vi "Setup V1.00.vi"(6 "Control Parameters Input":T1={"Grating Density"=enum."1200", "Offset"=0.0, "Save All Data in ONE file"=FALSE, "Auto Save Data"=FALSE, "Most recent saved file"=path "erererere", "Filename Prefix"="MyData", "Extension"=4, "Suffix"="", "Current Path"=path "/Volumes/DATA"} {"Extension" items=["DOS field", "\".001\",\".002\", ...", "001 (No dot)", "\".A\",\".B\", ...", "±Field", "pField nField", "Temperature", "User Defined"]; "Offset" format="%.2f"}, 7 "TempControl Input":bool[](array[boolean])=[TRUE, FALSE, FALSE, FALSE], 8 "Parameters#2 input":T2={"MaxBufferSize"=2, "Mag GPIB Address"=5, "Max Current (kA)"=36.0, "LTC-GPIB Address"="", "Temp Tolerance"=1.0} {"Temp Tolerance" format="%.2f"; "Max Current (kA)" format="%.2f"}, 9 "Parameters Input":T3={"Magnetic Field"=0.0, "Temperature"=0.0, "Exposure Time"=0.0, "Mag ID string"="", "User Name"="Albert Einstein", "Comments"="", "SaveComments?"=1, "X-Axis Unit"=1, "Delimiter"=0, "File Format"=0, "Sample Name"="Sample1"} {"File Format" items=["Macintosh (EOL: CR)", "Unix (EOL: LF)", "DOS/Windows (EOL: CR+LF)"]; "Delimiter" items=["TAB", "COMMA", "SPACE"]; "X-Axis Unit" items=["Point #", "nm", "eV", "meV", "cm-1"]; "SaveComments?" items=["Bare data only", "Saved in the Header Area", "Saved as a Parameter File"]; "Exposure Time" format="%.2f"; "Temperature" format="%.2f"; "Magnetic Field" format="%.2f"}) -> (0 "Control Parameters output":T1={"Grating Density"=enum."1200", "Offset"=0.0, "Save All Data in ONE file"=FALSE, "Auto Save Data"=FALSE, "Most recent saved file"=path "erererere", "Filename Prefix"="MyData", "Extension"=4, "Suffix"="", "Current Path"=path "/Volumes/DATA"} {"Extension" items=["DOS field", "\".001\",\".002\", ...", "001 (No dot)", "\".A\",\".B\", ...", "±Field", "pField nField", "Temperature", "User Defined"]; "Offset" format="%.2f"}, 1 "Parameters#2":T2={"MaxBufferSize"=2, "Mag GPIB Address"=5, "Max Current (kA)"=36.0, "LTC-GPIB Address"="", "Temp Tolerance"=1.0} {"Temp Tolerance" format="%.2f"; "Max Current (kA)" format="%.2f"}, 2 "TempControl":bool[](array[boolean])=[TRUE, FALSE, FALSE, FALSE], 3 "Parameters output":T3={"Magnetic Field"=0.0, "Temperature"=0.0, "Exposure Time"=0.0, "Mag ID string"="None", "User Name"="", "Comments"="", "SaveComments?"=1, "X-Axis Unit"=1, "Delimiter"=0, "File Format"=0, "Sample Name"="Sample1"} {"File Format" items=["Macintosh (EOL: CR)", "Unix (EOL: LF)", "DOS/Windows (EOL: CR+LF)"]; "Delimiter" items=["TAB", "COMMA", "SPACE"]; "X-Axis Unit" items=["Point #", "nm", "eV", "meV", "cm-1"]; "SaveComments?" items=["Bare data only", "Saved in the Header Area", "Saved as a Parameter File"]; "Exposure Time" format="%.2f"; "Temperature" format="%.2f"; "Magnetic Field" format="%.2f"}, 4 "McP off":bool=TRUE caption="McP on? output", 5 "CCD off":bool=TRUE caption="CCD on? output")   [LabVIEW 2021]
uses:
  Parameters#1.ctl
  Parameters#2.ctl
  Parameters_Control.ctl
  Globals and TypeDefs/Global Varibal Control.vi
  ExperimentLogGlobal.vi
panel:
  in  "Maximum BufferSize":u8=50 min=1 step=1
  in  "OpenUserProfile":bool
  out "Clock copy":string="1:26:45 AM"
  out "Clock":string="1:26:45 AM"
  in  "CCD on?":bool=TRUE caption="Off"
  out "CCD GPIB Address":u8=1 min=1 max=30
  in  "CCD LineSet?":bool caption="ldb,1,16,u,0,225,25,b,1,15;sdu,0,1024,1024;cl0;omrm;sron"
  in  "ChangeCounterPos?":bool
  in  "?":bool
  in  "LTC20 Cal Table?":bool
  in  "Hide?":bool
  out "GPIB Status":string
  in  "BusScan?":bool
  in  "Calibration":bool
  in  "X-Axis Unit":u16(ring)=1 items=["Point #", "nanometer (nm)", "electron volt (eV)", "Milli eV (meV)", "Wavenumber (cm-1)"]
  in  "SaveComments?":u16(ring)=1 items=["Bare data only", "Saved in the Header Area", "Saved as a Parameter File"]
  in  "Delimiter":u16(ring) items=["TAB", "COMMA", "SPACE"]
  in  "File Format":u16(ring) items=["Macintosh (EOL: CR)", "Unix (EOL: LF)", "DOS/Windows (EOL: CR+LF)"]
  in  "Max Current (kA)":dbl=36.0 caption="Maximum Current (kA)" format="%.2f"
  in  "User Name":string
  in  "Temp Tolerance":dbl=1.0 caption="Temperature Tolerance (if applicable)" format="%.2f"
  in  "LTC-GPIB Address":refnum<visa-resource-name> caption="GPIB Address"
  in  "Auto\nAdvance?":bool
  in  "Magneto\nCorrection?":bool
  in  "Mode:\nControl?":bool caption="Monitor"
  in  "LTC-20\nexist?":bool
  in  "SaveUserProfile":bool
  in  "Sample Name":string="Sample1"
  # "User Profile Panel"
  # "Magnet Control Panel"
  # "The Modem Port is reserved."
  # "Conductus LTC-20 Panel"
  # "Yes\n\nNo"
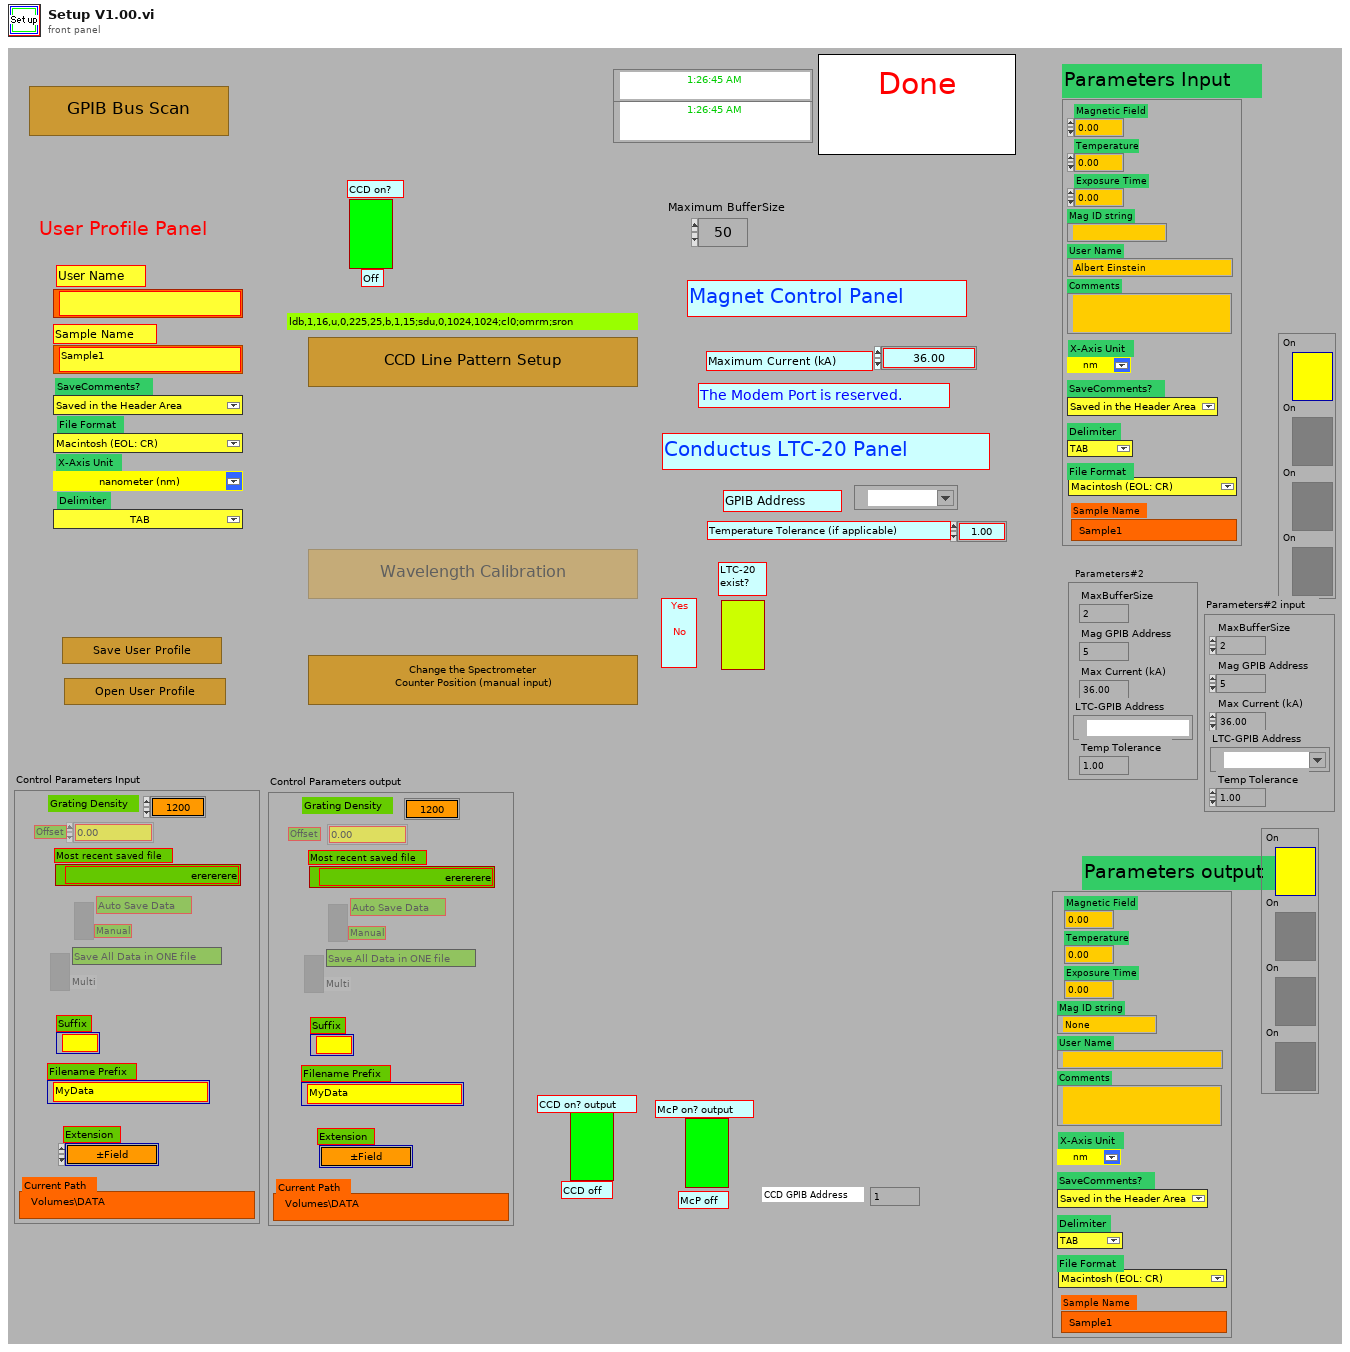
[diagram p1: front panel]
types:
  T1 = typedef "Parameters_Control.ctl" = cluster{"Grating Density":enum16{"150", "300", "600", "1200", "1800"}, "Offset":dbl, "Save All Data in ONE file":bool, "Auto Save Data":bool, "Most recent saved file":path, "Filename Prefix":string, "Extension":u16, "Suffix":string, "Current Path":path}
  T2 = typedef "Parameters#2.ctl" = cluster{"MaxBufferSize":i32, "Mag GPIB Address":i32, "Max Current (kA)":dbl, "LTC-GPIB Address":refnum<visa-resource-name>, "Temp Tolerance":dbl}
  T3 = typedef "Parameters#1.ctl" = cluster{"Magnetic Field":dbl, "Temperature":dbl, "Exposure Time":dbl, "Mag ID string":string, "User Name":string, "Comments":string, "SaveComments?":u16, "X-Axis Unit":u16, "Delimiter":u16, "File Format":u16, "Sample Name":string}
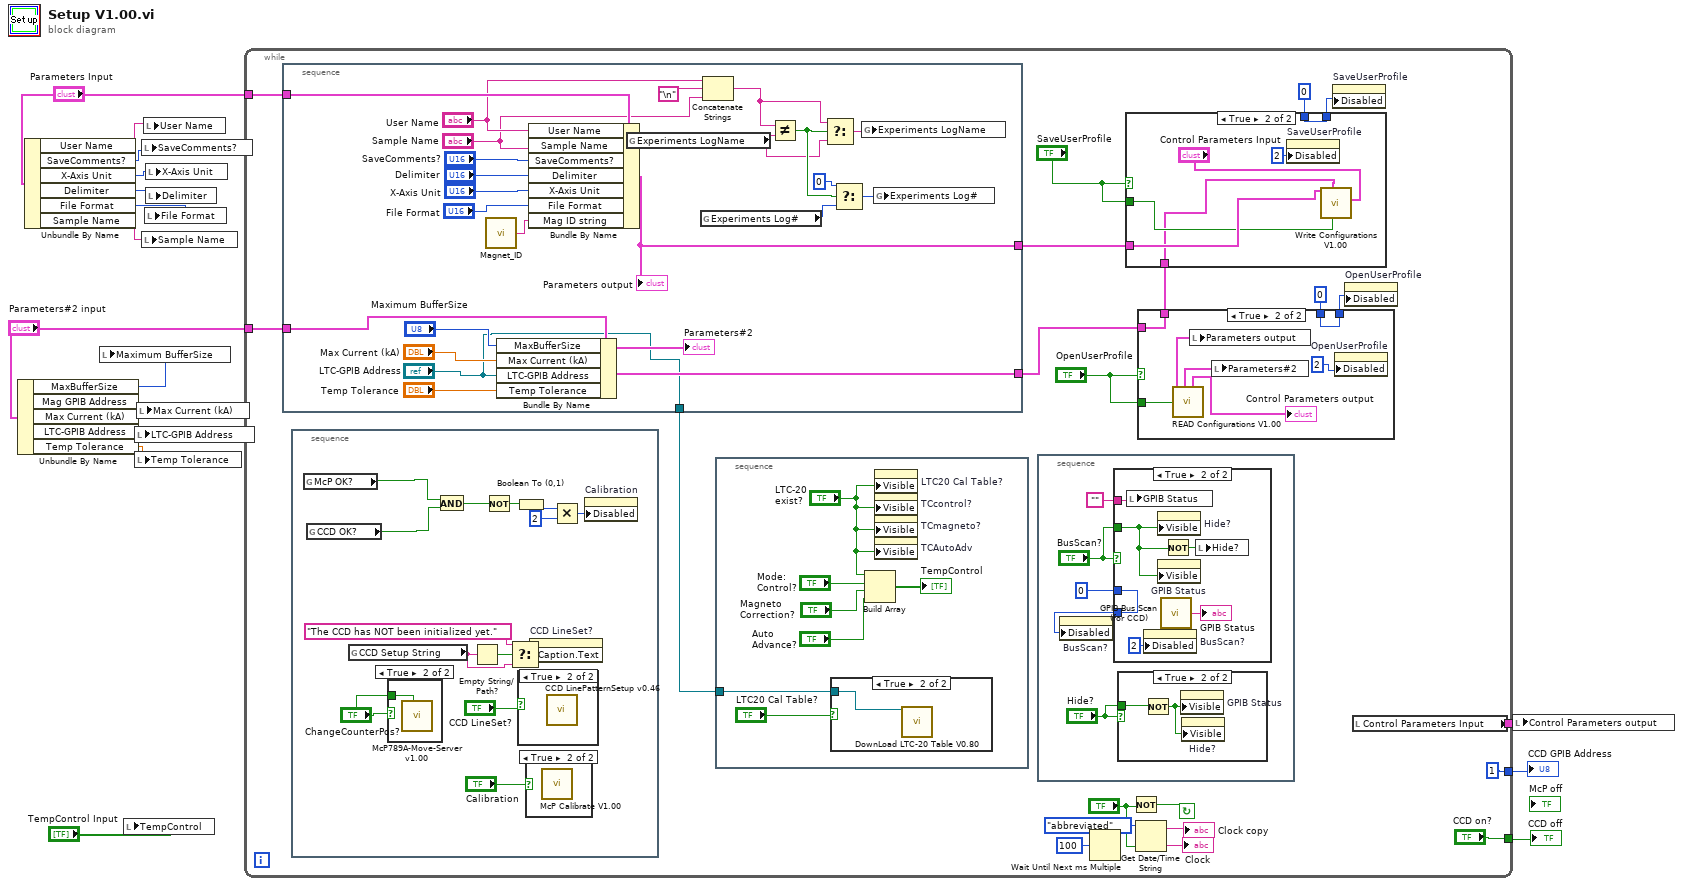
[diagram p0: block diagram]
diagram:
  n1 = Unbundle By Name("Parameters#2 input") -> ("MaxBufferSize"=w2:i32, "Max Current (kA)"=w7:dbl, "LTC-GPIB Address"=w6:refnum<visa-resource-name>, "Temp Tolerance"=w5:dbl)  [unwired: 1 out]
  n2 = Unbundle By Name("Parameters Input") -> ("User Name"=w9:string, "SaveComments?"=w10:u16, "X-Axis Unit"=w11:u16, "Delimiter"=w12:u16, "File Format"=w13:u16, "Sample Name"=w14:string)
  n3 = local write "Maximum BufferSize"(w2) -> ()
  n4 = local write "TempControl"("TempControl Input") -> ()
  n5 = local write "LTC-GPIB Address"(w6) -> ()
  n6 = local write "Temp Tolerance"(w5) -> ()
  n7 = local write "Max Current (kA)"(w7) -> ()
  n8 = local write "SaveComments?"(w10) -> ()
  n9 = local write "Sample Name"(w14) -> ()
  n10 = local write "User Name"(w9) -> ()
  n11 = local write "File Format"(w13) -> ()
  n12 = local write "X-Axis Unit"(w11) -> ()
  n13 = local write "Delimiter"(w12) -> ()
  n14 = while {
    tunnel: [w17] -> w1
    tunnel: ["CCD on?"] -> w3
    tunnel: "Parameters#2 input" -> [w33]
    tunnel: "Parameters Input" -> [w34]
    tunnel: [1] -> w16
    stop <- w37 continue-if-true
    n15 = stacked-sequence {
      tunnel: w34 -> [w96]
      tunnel: w33 -> [w82]
      tunnel: ["LTC-GPIB Address"] -> w27
      tunnel: [w84] -> w24
      tunnel: [w83] -> w23
      frame #0 {
        n16 = call "Magnet_ID.vi"() -> ("Cell"=w78:string)
        n17 = Bundle By Name(cluster=w82, "MaxBufferSize"="Maximum BufferSize", "Max Current (kA)"="Max Current (kA)", "LTC-GPIB Address"="LTC-GPIB Address", "Temp Tolerance"="Temp Tolerance") -> (w83:T2)
        "Parameters#2" <- w83
        n18 = Bundle By Name(cluster=w96, "User Name"="User Name", "Sample Name"="Sample Name", "SaveComments?"="SaveComments?", "Delimiter"="Delimiter", "X-Axis Unit"="X-Axis Unit", "File Format"="File Format", "Mag ID string"=w78) -> (w84:T3)
        "Parameters output" <- w84
        n19 = global read "ExperimentLogGlobal.vi" "Experiments LogName"() -> (w86:string)
        n20 = global read "ExperimentLogGlobal.vi" "Experiments Log#"() -> (w87:u32)
        n21 = Concatenate Strings("User Name", "\n", "Sample Name") -> (w91:string)
        n22 = Not Equal?(x=w91, y=w86) -> (x != y?=w90:bool)
        n23 = Select(t=w91, s=w90, f=w86) -> (s? t:f=w85:string)
        n24 = Select(t=0, s=w90, f=w87) -> (s? t:f=w88:u32)
        n25 = global write "ExperimentLogGlobal.vi" "Experiments LogName"(w85) -> ()
        n26 = global write "ExperimentLogGlobal.vi" "Experiments Log#"(w88) -> ()
      }
    }
    n27 = stacked-sequence {
      frame #0 {
        n28 = global read "Global Varibal Control.vi" "McP OK?"() -> (w55:bool)
        n29 = global read "Global Varibal Control.vi" "CCD OK?"() -> (w54:bool)
        n30 = global read "Global Varibal Control.vi" "CCD Setup String"() -> (w63:string)
        n31 = case shown="True" "ChangeCounterPos?" {
          tunnel: "ChangeCounterPos?" -> [_ w68]
          frame False {
          }
          frame True {
            n32 = call "McP789A-Move-Server v1.00.vi"("Change Counter Position Manually"=w68) -> ()  [unwired: 7 in, 3 out]
          }
        }
        n33 = And(x=w55, y=w54) -> (x .and. y?=w58:bool)
        n34 = Empty String/Path?(string/path=w63) -> (empty?=w65:bool)
        n35 = Not(x=w58) -> (.not. x?=w61:bool)
        n36 = Select(t="The CCD has NOT been initialized yet.", s=w65, f=w63) -> (s? t:f=w62:string)
        n37 = Boolean To (0,1)(Boolean=w61) -> (0, 1=w60:i16)
        n38 = case shown="True" "CCD LineSet?" {
          frame False {
          }
          frame True {
            n39 = call "CCD LinePatternSetup v0.46.vi"() -> ()  [unwired: 9 in, 2 out]
          }
        }
        n40 = case shown="True" "Calibration" {
          frame False {
          }
          frame True {
            n41 = call "McP Calibrate V1.00.vi"() -> ()  [unwired: 1 in]
          }
        }
        n42 = property on="CCD LineSet?" class="Bool"("Caption.Text"=w62) -> ()  [unwired: 2 in, 2 out]
        n43 = Multiply(x=w60, y=i16 2) -> (x*y=w57:i16)
        n44 = property on="Calibration" class="Bool"("Disabled"=w57) -> ()  [unwired: 2 in, 2 out]
      }
    }
    n45 = stacked-sequence {
      tunnel: w27 -> [w69]
      frame #0 {
        n46 = case shown="True" "LTC20 Cal Table?" {
          tunnel: w69 -> [_ w76]
          frame False {
          }
          frame True {
            n47 = call "DownLoad LTC-20 Table V0.80.vi"("LTC-20 GPIB"=w76) -> ()  [unwired: 16 in, 3 out]
          }
        }
        n48 = Build Array("LTC-20\nexist?", "Mode:\nControl?", "Magneto\nCorrection?", "Auto\nAdvance?") -> (→"TempControl":bool[])
        n49 = property on="LTC20 Cal Table?" class="Bool"("Visible"="LTC-20\nexist?") -> ()  [unwired: 2 in, 2 out]
        n50 = property on="TCcontrol?" class="Bool (strict)"("Visible"="LTC-20\nexist?") -> ()  [unwired: 2 in, 2 out]
        n51 = property on="TCmagneto?" class="Bool (strict)"("Visible"="LTC-20\nexist?") -> ()  [unwired: 2 in, 2 out]
        n52 = property on="TCAutoAdv" class="Bool (strict)"("Visible"="LTC-20\nexist?") -> ()  [unwired: 2 in, 2 out]
      }
    }
    n53 = stacked-sequence {
      frame #0 {
        n54 = case shown="True" "BusScan?" {
          tunnel: "" -> [_ w112]
          tunnel: "BusScan?" -> [_ w110]
          tunnel: [w107 w108] -> w100
          tunnel: u8 0 ("Write Attribute") -> [w107 w108]
          frame False {
          }
          frame True {
            n55 = local write "GPIB Status"(w112) -> ()
            n56 = property on="BusScan?" class="Bool"("Disabled"=u8 2 ("Write Attribute")) -> ()  [unwired: 2 in, 2 out]
            n57 = property on="Hide?" class="Bool (strict)"("Visible"=w110) -> ()  [unwired: 2 in, 2 out]
            n58 = property on="GPIB Status" class="Str"("Visible"=w110) -> ()  [unwired: 2 in, 2 out]
            n59 = call "GPIB Bus Scan (for CCD).vi"() -> (0:→"GPIB Status":string)  [unwired: 1 in]
            n60 = Not(x=w110) -> (.not. x?=w111:bool)
            n61 = local write "Hide?"(w111) -> ()
          }
        }
        n62 = property on="BusScan?" class="Bool"("Disabled"=w100) -> ()  [unwired: 2 in, 2 out]
        n63 = case shown="True" "Hide?" {
          tunnel: "Hide?" -> [_ w106]
          frame False {
          }
          frame True {
            n64 = Not(x=w106) -> (.not. x?=w105:bool)
            n65 = property on="GPIB Status" class="Str"("Visible"=w105) -> ()  [unwired: 2 in, 2 out]
            n66 = property on="Hide?" class="Bool (strict)"("Visible"=w105) -> ()  [unwired: 2 in, 2 out]
          }
        }
      }
    }
    n67 = Wait Until Next ms Multiple(millisecond multiple=u32 100) -> ()  [unwired: 1 out]
    n68 = Not(x="?") -> (.not. x?=w37:bool)
    n69 = Get Date/Time String(date format (0)=enum16{"short", "long", "abbreviated"}."abbreviated", want seconds? (F)="?") -> (date string=→"Clock copy":string, time string=→"Clock":string)  [unwired: 1 in]
    n70 = case shown="True" "OpenUserProfile" {
      tunnel: "OpenUserProfile" -> [_ w43]
      tunnel: [w39 w42] -> w22
      tunnel: w23 -> [w39 w42]
      tunnel: [w38 w41] -> w19
      tunnel: u8 0 ("Write Attribute") -> [w38 w41]
      frame False {
      }
      frame True {
        n71 = call "READ Configurations V1.00.vi"("OpenParameters(T)orDataBuffers(F)"=w43) -> ("Parameters"=w45:T3, "Parameters#2"=w44:T2, "Control Parameters"=→"Control Parameters output":T1)  [unwired: 2 in, 4 out]
        n72 = local write "Parameters output"(w45) -> ()
        n73 = local write "Parameters#2"(w44) -> ()
        n74 = property on="OpenUserProfile" class="Bool"("Disabled"=u8 2 ("Write Attribute")) -> ()  [unwired: 2 in, 2 out]
      }
    }
    n75 = case shown="True" "SaveUserProfile" {
      tunnel: "SaveUserProfile" -> [_ w51]
      tunnel: w24 -> [_ w52]
      tunnel: w22 -> [_ w50]
      tunnel: [w47 w48] -> w21
      tunnel: u8 0 ("Write Attribute") -> [w47 w48]
      frame False {
      }
      frame True {
        n76 = property on="SaveUserProfile" class="Bool"("Disabled"=u8 2 ("Write Attribute")) -> ()  [unwired: 2 in, 2 out]
        n77 = call "Write Configurations V1.00.vi"("Control Parameters"="Control Parameters Input", "SaveParameters(T)/DataBuffer(F)?"=w51, "Parameters#2"=w50, "Parameters"=w52) -> ()  [unwired: 6 in, 1 out]
      }
    }
    n78 = property on="SaveUserProfile" class="Bool"("Disabled"=w21) -> ()  [unwired: 2 in, 2 out]
    n79 = property on="OpenUserProfile" class="Bool"("Disabled"=w19) -> ()  [unwired: 2 in, 2 out]
    n80 = local read "Control Parameters Input"() -> (w17:T1)
  }
  "CCD GPIB Address" <- w16
  "CCD off" <- w3
  n81 = local write "Control Parameters output"(w1) -> ()
